vi "PRIME Detector Read Final Reduced Frames.vi"(11 "Final Reduced Frame":T2) -> (3 "Images":T1[](array[typedef]))   [LabVIEW 2024, in "PRIME Detector.lvclass"]
uses:
  PRIME Detector.lvclass
  Detector Image typedef cluster.ctl
  Detector Class.lvclass
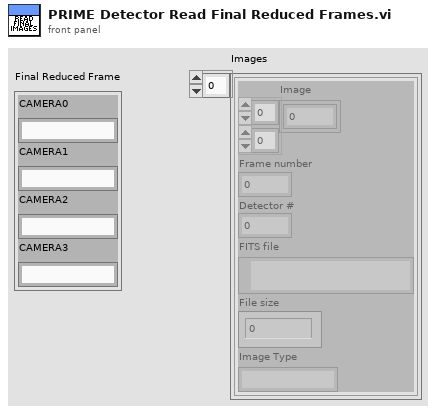
[diagram p1: front panel]
types:
  T1 = typedef "Detector Class.lvclass/Detector Image typedef cluster.ctl" = cluster{"Image":sgl[][], "Frame number":i32, "Detector #":u16, "FITS file":path, "File size":i64, "Image Type":string}
  T2 = cluster{"CAMERA0":string, "CAMERA1":string, "CAMERA2":string, "CAMERA3":string}
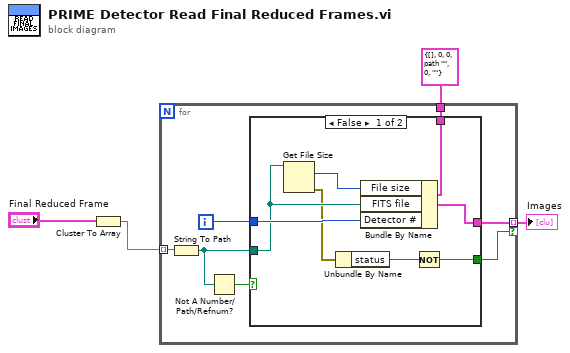
[diagram p0: block diagram]
diagram:
  n1 = Cluster To Array(cluster="Final Reduced Frame") -> (array=w3:string[])
  n2 = for {
    tunnel: w3 -> [w11] mode=indexing
    tunnel: T1 {"Image"=[], "Frame number"=0, "Detector #"=0, "FITS file"=path "", "File size"=0, "Image Type"=""} ("Image Data") -> [w10]
    tunnel: [w9] -> w1 mode=indexing if=w5
    i -> [w8]
    n3 = String To Path(string=w11) -> (path=w7:path)
    n4 = Not A Number/Path/Refnum?(number/path/refnum=w7) -> (NaN/Path/Refnum?=w6:bool)
    n5 = case shown="False" w6 {
      tunnel: w10 -> [w19 w20]
      tunnel: [w18 w20] -> w9
      tunnel: w8 -> [w17 _]
      tunnel: w7 -> [w16 _]
      tunnel: [w12 _] -> w5
      frame False {
        n6 = Get File Size(file=w16) -> (size (in bytes)=w15:i64, 0:w14:errorcluster)  [unwired: 1 in, 1 out]
        n7 = Unbundle By Name(w14) -> ("status"=w13:bool)
        n8 = Bundle By Name(cluster=w19, "File size"=w15, "FITS file"=w16, "Detector #"=w17) -> (w18:T1)
        n9 = Not(x=w13) -> (.not. x?=w12:bool)
      }
      frame True {
      }
    }
  }
  "Images" <- w1
